vi "fpga.top.vi"(9 "data_valid_in":bool, 10 "end_of_frame_in":bool, 11 "data_in":u8) -> (1 "tvalid":bool, 2 "tlast":bool, 3 "tdata":u8)   [LabVIEW 2022 SP3]
uses:
  <vilib>/Platform/TimedLoop/XDataNode/XDataNode.xnode
  <vilib>/Platform/TimedLoop/XDataNode/nitl_modes.ctl
  <vilib>/Platform/TimedLoop/XDataNode/XDNodeRunTimeDep.lvlib
  <vilib>/Platform/TimedLoop/XDataNode/wakeup.ctl
  <vilib>/Platform/TimedLoop/XDataNode/timing_clust.ctl
  <vilib>/rvi/DataTransferAndStorage/Container/XNode/niFpgaContainer.xnode
  <vilib>/rvi/LocalResourceManager/LocalResourceManager.xnode
  <vilib>/rvi/FIFO/Fifo_Resource/niFpgaFifoEmulationRefIn.vi
  <vilib>/rvi/DataTransferAndStorage/Container/Common/niFpgaContainerGetUniqueNameForEmu.vi
  <vilib>/rvi/DataTransferAndStorage/Container/Common/niFpgaContainerSetEmuInfo.vi
  <vilib>/rvi/eio/common/nirviEmuReportErrorAndStop.vi
  <instrlib>/_niInstr/Network/Types/v1/IPv4 Address.ctl
  <instrlib>/_niInstr/Network/Types/v1/niInstr Network Types v1.lvlib
  <instrlib>/_niInstr/Network/Types/v1/MAC Address.ctl
panel:
  in  "MAC Address":T1=[0, 10, 53, 0, 1, 2] format="%.0x"
  in  "IP Address":T2=[192, 168, 1, 60]
  in  "Dest Port":u16=6001
  out "out_2":bool
  out "out_1":bool
  in  "in_2":bool
  in  "in_1":bool
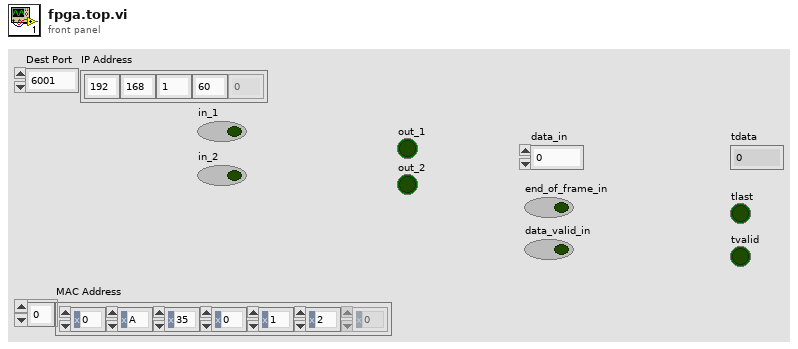
[diagram p1: front panel]
types:
  T1 = typedef "niInstr Network Types v1.lvlib/MAC Address.ctl" = u8[]
  T2 = typedef "niInstr Network Types v1.lvlib/IPv4 Address.ctl" = u8[]
  T3 = typedef "XDNodeRunTimeDep.lvlib/timing_clust.ctl" = cluster{"Expected End [f-1]":u64, "Actual End [f-1]":u64, "Finished Late? [f-1]":bool, "Expected End [i-1]":u64, "Actual End [i-1]":u64, "Finished Late? [i-1]":bool, "Expected Start [i]":u64, "Actual Start [i]":u64, "Expected Start [f]":u64, "Actual Start [f]":u64, "Source Name":string, "Structure Name":string, "Period":i64, "Deadline":i64, "Offset":i64, "Start":i64, "Priority":i32, "Timeout":i32, "Mode":T4, "Wakeup Reason":T5, "Error":errorcluster, "Source Type":string, "Secondary Source Type":string, "Global End Time":u64, "Global Start Time":u64, "Frame Duration":u64, "Iteration Duration":u64, "Assigned CPU":i32, "I/O Scan Engine Mode":u32}
  T4 = typedef "XDNodeRunTimeDep.lvlib/nitl_modes.ctl" = enum32{"No Change", "Process missed periods, maintain original phase", "Discard missed periods, maintain original phase", "Process missed periods, ignore original phase", "Discard missed periods, ignore original phase"}
  T5 = typedef "XDNodeRunTimeDep.lvlib/wakeup.ctl" = enum32{"Normal", "Aborted", "Asynchronous wakeup", "Timing source error", "Timed loop error", "Timeout"}
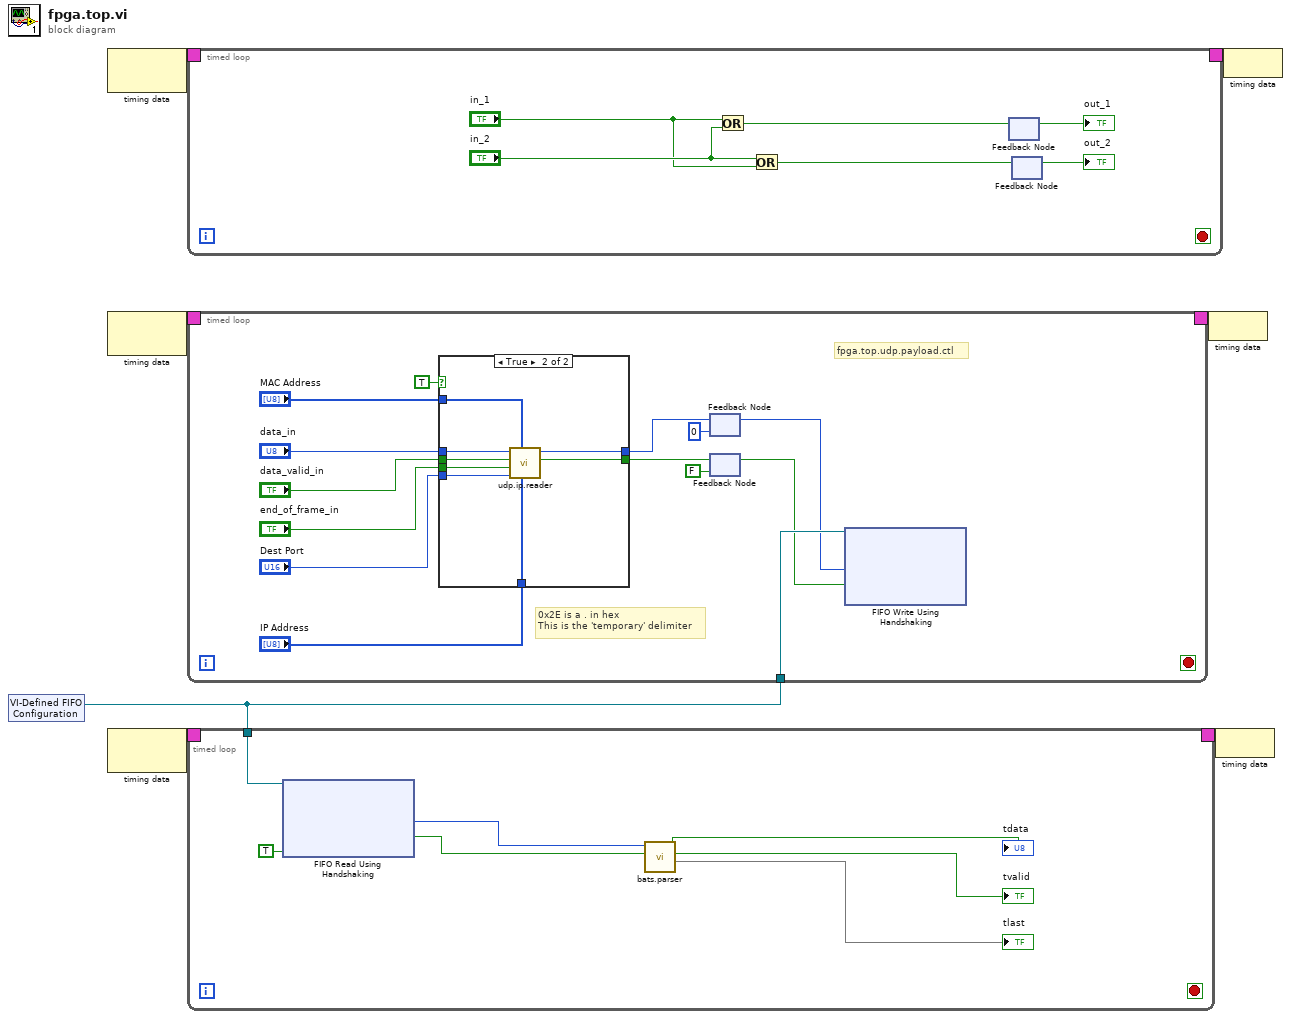
[diagram p0: block diagram]
diagram:
  n1 = xnode "VI-Defined FIFO Configuration"() -> ("FIFO Out"=w1:refnum<k21>)
  n2 = node-c288() -> (w7:T3)  [unwired: 1 in]
  n3 = node-c288() -> (w5:T3)  [unwired: 1 in]
  n4 = node-c288() -> (w3:T3)  [unwired: 1 in]
  n5 = timed-loop {
    timing: w7 -> [_]
    timing-out: [_] -> w6
    stop <- _ stop-if-true
    n6 = Or(x="in_1", y="in_2") -> (x .or. y?=w13:bool)
    n7 = Or(x="in_2", y="in_1") -> (x .or. y?=w12:bool)
    n8 = feedback-in #1(w13) -> ()
    n9 = feedback #1() -> (→"out_1":bool)  [unwired: 1 in]
    n10 = feedback-in #2(w12) -> ()
    n11 = feedback #2() -> (→"out_2":bool)  [unwired: 1 in]
  }
  n12 = timed-loop {
    timing: w5 -> [_]
    timing-out: [_] -> w4
    tunnel: w1 -> [w18]
    stop <- _ stop-if-true
    # "fpga.top.udp.payload.ctl"
    # "0x2E is a . in hex\nThis is the 'temporary' delimiter"
    n13 = case shown="True" TRUE {
      tunnel: "data_in" -> [w31 w39]
      tunnel: "data_valid_in" -> [w30 w38]
      tunnel: "end_of_frame_in" -> [_ w37]
      tunnel: "MAC Address" -> [_ w36]
      tunnel: "Dest Port" -> [_ w35]
      tunnel: "IP Address" -> [_ w34]
      tunnel: [w30 w33] -> w23
      tunnel: [w31 w32] -> w22
      frame False {
      }
      frame True {
        n14 = call "udp.ip.reader.vi"("IP Address"=w34, "MAC Address"=w36, "Dest Port"=w35, "end_of_frame"=w37, "data_valid"=w38, "data"=w39) -> ("udp_data valid_out"=w33:bool, "udp_data_out"=w32:u8)  [unwired: 3 in, 1 out]
      }
    }
    n15 = feedback-in #3(w22) -> ()
    n16 = feedback #3(u8 0 ("udp_data_out")) -> (w16:u8)
    n17 = feedback-in #4(w23) -> ()
    n18 = feedback #4(FALSE ("udp_data valid_out")) -> (w17:bool)
    n19 = xnode "FIFO Write Using Handshaking"("Element"=w16, "Input Valid"=w17, "FIFO In"=w18) -> ()  [unwired: 2 out]
  }
  n20 = timed-loop {
    timing: w3 -> [_]
    timing-out: [_] -> w2
    tunnel: w1 -> [w48]
    stop <- _ stop-if-true
    n21 = xnode "FIFO Read Using Handshaking"("Ready for Output"=TRUE, "FIFO In"=w48) -> ("Element"=w42:u8, "Output Valid"=w46:bool)  [unwired: 1 out]
    n22 = call "bats.parser.vi"("data.valid"=w46, "data"=w42) -> (1:→"tlast", "Ready.for.Configuration.Input"=→"tvalid":bool, "Ready.for.Udp.Input"=→"tdata":bool)  [unwired: 7 in]
  }
  n23 = node-c288(w4) -> ()
  n24 = node-c288(w2) -> ()
  n25 = node-c288(w6) -> ()
